vi "NT Bind Controls to SmartDashboard.vi"(6 "Update Time (ms)":i32=100, 8 "Client Name":string="Dashboard", 9 "Path Prefix":string="SmartDashboard", 10 "Bound Control Refs":refnum<vi>[](array[refnum])) -> ()   [LabVIEW 2025]
doc: "Place this VI in the Dashboard or other client applications so that it can run in parallel with the other tasks. Provide the robot IP address so that it can know where to find the server. This starts the NT Client automatically.\n\nCombine the path prefix and control name to construct entry names. Bind controls and indicators to a SmartDashboard or Network Table entry with the matching name. Controls and Indicators will be updated each time the table entriy of the same name changes. Table entries will be updated each time the control changes value."
uses:
  24746e4c-8412-4618-8ce7-7cb261ceb86e.vi
  2f59ec2f-4d8f-49a6-9fcf-95b307e91e62.vi
  24746e4c-8412-4618-8ce7-7cb261ceb86e.vi/d4db2432-cc9c-482c-8957-dac855435ef6.vi
  24746e4c-8412-4618-8ce7-7cb261ceb86e.vi/86fbf154-bd7b-49a2-8ab2-a837b2a95f24.vi
  24746e4c-8412-4618-8ce7-7cb261ceb86e.vi/3b95b01e-1ec2-4565-bcd9-7606a5281010.vi
  24746e4c-8412-4618-8ce7-7cb261ceb86e.vi/96a08935-737a-44b2-979c-a81d56408f7e.vi
  24746e4c-8412-4618-8ce7-7cb261ceb86e.vi/d4db2432-cc9c-482c-8957-dac855435ef6.vi/6eaecd13-6e48-4772-a921-b51ebdf84d88.vi
  24746e4c-8412-4618-8ce7-7cb261ceb86e.vi/d4db2432-cc9c-482c-8957-dac855435ef6.vi/d2d5f2b7-06f4-47f6-971c-049c3fdbb653.vi
  24746e4c-8412-4618-8ce7-7cb261ceb86e.vi/3b95b01e-1ec2-4565-bcd9-7606a5281010.vi/6eaecd13-6e48-4772-a921-b51ebdf84d88.vi
  24746e4c-8412-4618-8ce7-7cb261ceb86e.vi/3b95b01e-1ec2-4565-bcd9-7606a5281010.vi/d2d5f2b7-06f4-47f6-971c-049c3fdbb653.vi
  24746e4c-8412-4618-8ce7-7cb261ceb86e.vi/96a08935-737a-44b2-979c-a81d56408f7e.vi/6eaecd13-6e48-4772-a921-b51ebdf84d88.vi
  24746e4c-8412-4618-8ce7-7cb261ceb86e.vi/96a08935-737a-44b2-979c-a81d56408f7e.vi/d2d5f2b7-06f4-47f6-971c-049c3fdbb653.vi
  <vilib>/Comparison/Less/Less Functor/Less Functor.lvclass
  <vilib>/Comparison/Equal/Equal Functor/Equal Functor.lvclass
panel:
  out "Value out":variant
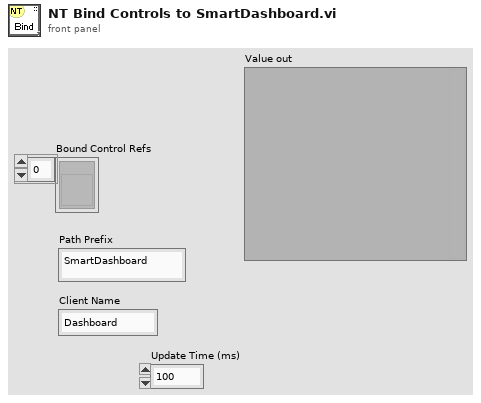
[diagram p1: front panel]
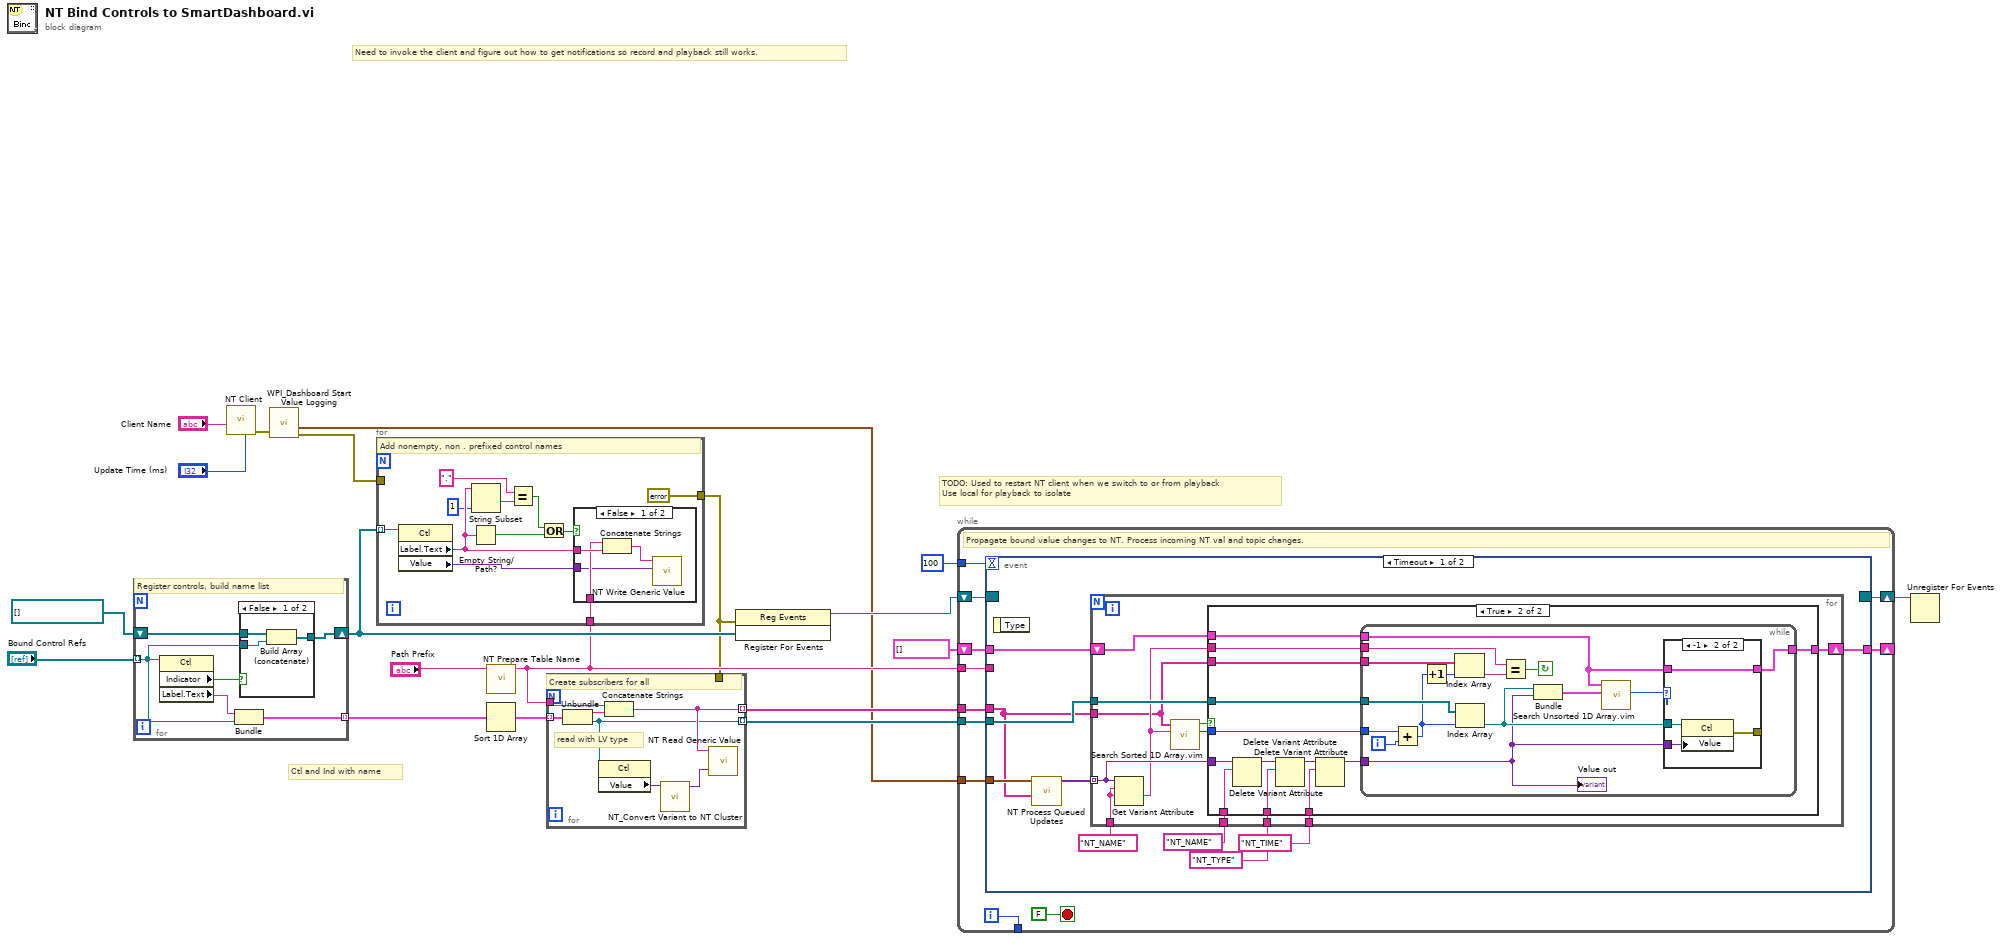
[diagram p0: block diagram]
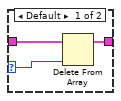
[diagram p3: hidden frame]
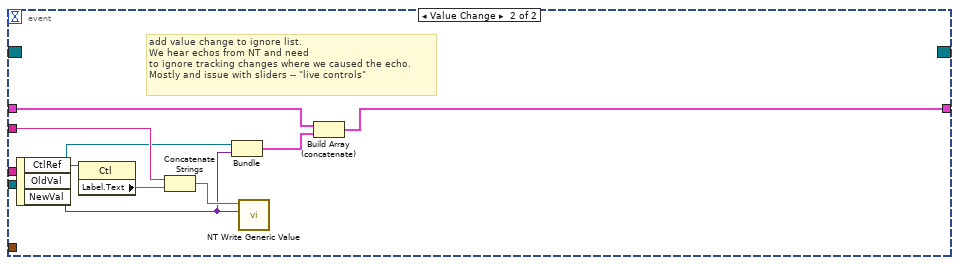
[diagram p4: hidden frame]
diagram:
  # "TODO: Used to restart NT client when we switch to or from playback\nUse local for playback to isolate"
  # "Need to invoke the client and figure out how to get notifications so record and playback still works."
  # "Ctl and Ind with name"
  n1 = for {
    tunnel: "Bound Control Refs" -> [w22] mode=indexing
    shift-right: [w23] -> w14
    shift-left: refnum<vi>[] [] -> [w24]
    tunnel: [w20] -> w18 mode=indexing
    # "Register controls, build name list"
    n2 = property class="Ctl"(reference=w22) -> ("Indicator"=w25:bool, "Label.Text"=w21:string)  [unwired: 1 in, 2 out]
    n3 = Bundle("Label.Text"=w21, w22) -> (w20:cluster{"Label.Text":string, refnum<vi>})  [unwired: 1 in]
    n4 = case shown="False" w25 {
      tunnel: w22 -> [w28 _]
      tunnel: w24 -> [w27 w29]
      tunnel: [w26 w29] -> w23
      frame False {
        n5 = Build Array (concatenate)(w27, w28) -> (w26:refnum<vi>[])
      }
      frame True {
      }
    }
  }
  n6 = call <vilib>:"NT Client.vi"("Update Time"="Update Time (ms)", "Client Name"="Client Name") -> ("error out"=w3:errorcluster)  [unwired: 9 in]
  n7 = call <vilib>:"WPI_Dashboard Start Value Logging.vi"("error in (no error)"=w3) -> ("error out"=w2:errorcluster, "handles"=w4:cluster{"poller":u32, "overAll Listener":u32})  [unwired: 9 in]
  n8 = call <vilib>:"NT Prepare Table Name.vi"("Table Prefix"="Path Prefix") -> ("Prefixed Name"=w12:string)  [unwired: 10 in]
  n9 = for {
    tunnel: w14 -> [w40] mode=indexing
    tunnel: w12 -> [w38]
    tunnel: [errorcluster {"status"=FALSE, "code"=0, "source"=""} ("error out")] -> w5
    tunnel: w2 -> [_]
    # "Add nonempty, non . prefixed control names"
    n10 = property class="Ctl"(reference=w40) -> ("Label.Text"=w36:string, "Value"=w39:variant)  [unwired: 1 in, 2 out]
    n11 = Empty String/Path?(string/path=w36) -> (empty?=w37:bool)
    n12 = String Subset(string=w36, length (rest)=1) -> (substring=w34:string)  [unwired: 1 in]
    n13 = Equal?(x=".", y=w34) -> (x = y?=w32:bool)
    n14 = Or(x=w32, y=w37) -> (x .or. y?=w31:bool)
    n15 = case shown="False" w31 {
      tunnel: w39 -> [w41 _]
      tunnel: w36 -> [w44 _]
      tunnel: w38 -> [w42 _]
      frame False {
        n16 = Concatenate Strings(w42, w44) -> (w43:string)
        n17 = call <vilib>:"NT Write Generic Value.vi"("Variant"=w41, "Name"=w43) -> ()  [unwired: 9 in, 1 out]
      }
      frame True {
      }
    }
  }
  n18 = Sort 1D Array(array=w18) -> (sorted array=w17:cluster{"Label.Text":string, refnum<vi>}[])
  n19 = for {
    tunnel: w17 -> [w51] mode=indexing
    tunnel: [w48] -> w16 mode=indexing
    tunnel: [w47] -> w6 mode=indexing
    tunnel: w12 -> [w49]
    tunnel: w5 -> [_]
    # "read with LV type"
    # "Create subscribers for all"
    n20 = Unbundle(w51) -> ("Label.Text"=w50:string, w47:refnum<vi>)
    n21 = property class="Ctl"(reference=w47) -> ("Value"=w46:variant)  [unwired: 1 in, 2 out]
    n22 = Concatenate Strings(w49, w50) -> (w48:string)
    n23 = call <vilib>:"NT_Convert Variant to NT Cluster.vi"("NewVal"=w46) -> ("Value out"=w45:variant)  [unwired: 9 in, 1 out]
    n24 = call <vilib>:"NT Read Generic Value.vi"("type variant"=w45, "name"=w48) -> ()  [unwired: 8 in, 2 out]
  }
  n25 = register-events(error in=w5, w14) -> (reference out=w10:refnum<event-registration>)  [unwired: 1 in, 1 out]
  n26 = while {
    tunnel: w16 -> [w62]
    tunnel: w6 -> [w61]
    tunnel: w12 -> [w60]
    tunnel: [w59] -> _
    shift-right: [w58] -> w9
    shift-left: w10 -> [w56]
    tunnel: 100 -> [w57]
    tunnel: w4 -> [w54]
    shift-right: [w52] -> _
    shift-left: cluster{"CtlRef":refnum<vi>, "NewVal":variant}[] [] -> [w53]
    i -> [w59]
    stop <- FALSE ("Automatic restart") stop-if-true
    # "Propagate bound value changes to NT. Process incoming NT val and topic changes."
    n27 = event shown="[0] Timeout" {
      selector: w56 -> [_ _]
      dyn-events: [_ _] -> w58
      timeout: w57 -> [_ _]
      tunnel: w62 -> [w63 _]
      tunnel: w61 -> [w71 _]
      tunnel: w60 -> [_ w126]
      tunnel: w54 -> [w65 _]
      tunnel: w53 -> [w70 w123]
      tunnel: [w69 w121] -> w52
      event Timeout {
        n28 = event-data() -> ()  [unwired: 1 in, 1 out]
        n29 = call <vilib>:"NT Process Queued Updates.vi"("Bound Names"=w63, "handles"=w65) -> ("Updates"=w64:variant[])  [unwired: 9 in]
        n30 = for {
          tunnel: w63 -> [w78]
          tunnel: w64 -> [w83] mode=indexing
          tunnel: "NT_NAME" ("String") -> [w84]
          tunnel: w71 -> [w82]
          shift-right: [w76] -> w69
          shift-left: w70 -> [w77]
          tunnel: "NT_NAME" ("String") -> [w75]
          tunnel: "NT_TYPE" ("String") -> [w74]
          tunnel: "NT_TIME" ("String") -> [w73]
          n31 = Get Variant Attribute(Variant=w83, name=w84, default value (empty Variant)=w84) -> (value=w81:string)  [unwired: 1 in, 3 out]
          n32 = call "Search Sorted 1D Array.vim"("element"=w81, "sorted 1D array"=w78) -> ("nearest index"=w79:i32, "found?"=w80:bool)  [unwired: 8 in]
          n33 = case shown="True" w80 {
            tunnel: w83 -> [_ w92]
            tunnel: w81 -> [_ w95]
            tunnel: w82 -> [_ w98]
            tunnel: w79 -> [_ w97]
            tunnel: w78 -> [_ w96]
            tunnel: w77 -> [w85 w94]
            tunnel: [w85 w93] -> w76
            tunnel: w75 -> [_ w91]
            tunnel: w74 -> [_ w89]
            tunnel: w73 -> [_ w86]
            frame False {
            }
            frame True {
              n34 = Delete Variant Attribute(6:w91, 7:w92) -> (3:w90:variant)  [unwired: 1 in, 2 out]
              n35 = Delete Variant Attribute(6:w89, 7:w90) -> (3:w88:variant)  [unwired: 1 in, 2 out]
              n36 = Delete Variant Attribute(6:w86, 7:w88) -> (3:w87:variant)  [unwired: 1 in, 2 out]
              n37 = while {
                tunnel: w98 -> [w112]
                tunnel: w97 -> [w109]
                tunnel: w87 -> [w100]
                tunnel: w96 -> [w111]
                tunnel: w95 -> [w106]
                tunnel: w94 -> [w99]
                tunnel: [w101] -> w93
                i -> [w113]
                stop <- w105 continue-if-true
                n38 = Add(x=w109, y=w113) -> (x+y=w108:i32)
                n39 = Increment(x=w108) -> (x+1=w110:i32)
                n40 = Index Array(array=w111, index=w110) -> (element=w107:string)
                n41 = Index Array(array=w112, index=w108) -> (element=w104:refnum<vi>)
                n42 = Equal?(x=w106, y=w107) -> (x = y?=w105:bool)
                n43 = Bundle(w104, w100) -> (w103:cluster{refnum<vi>, variant})  [unwired: 1 in]
                n44 = call "Search Unsorted 1D Array.vim"("element"=w103, "unsorted 1D array"=w99) -> ("index of element"=w102:i32)  [unwired: 9 in]
                n45 = case shown="-1" w102 {
                  selector: w102 -> [w115 _]
                  tunnel: w104 -> [_ w120]
                  tunnel: w100 -> [_ w119]
                  tunnel: [_ w118] -> _
                  tunnel: w99 -> [w116 w117]
                  tunnel: [w114 w117] -> w101
                  frame Default {
                    n46 = Delete From Array(array=w116, index=w115) -> (array with subset deleted=w114:cluster{"CtlRef":refnum<vi>, "NewVal":variant}[])  [unwired: 1 in, 1 out]
                  }
                  frame -1 {
                    n47 = property class="Ctl"(reference=w120, "Value"=w119) -> (error out=w118:errorcluster)  [unwired: 1 in, 1 out]
                  }
                }
                "Value out" <- w100
              }
            }
          }
        }
      }
      event Value Change {
        # "add value change to ignore list.\nWe hear echos from NT and need\nto ignore tracking changes where we caused the echo.\nMostly and issue with sliders -- \"live controls\""
        n48 = event-data() -> ("CtlRef"=w125:refnum<vi>, "NewVal"=w124:variant)  [unwired: 1 in, 1 out]
        n49 = property class="Ctl"(reference=w125) -> ("Label.Text"=w128:string)  [unwired: 1 in, 2 out]
        n50 = Concatenate Strings(w126, w128) -> (w127:string)
        n51 = Bundle("CtlRef"=w125, "NewVal"=w124) -> (w122:cluster{"CtlRef":refnum<vi>, "NewVal":variant})  [unwired: 1 in]
        n52 = call <vilib>:"NT Write Generic Value.vi"("Variant"=w124, "Name"=w127) -> ()  [unwired: 9 in, 1 out]
        n53 = Build Array (concatenate)(w123, w122) -> (w121:cluster{"CtlRef":refnum<vi>, "NewVal":variant}[])
      }
    }
  }
  n54 = Unregister For Events(event registration refnum=w9) -> ()  [unwired: 1 in, 1 out]
